vi "Untitled 1.vi"() -> ()   [LabVIEW 2018]
uses:
  <vilib>/imath/engines/lvmath/Plug In/_Char/NIMS_CH_character datatype.ctl
  <vilib>/imath/engines/lvmath2/RunTimeEngine/Managers/WorkSpace/UID Generator.vi
  <vilib>/imath/engines/lvmath2/RunTimeEngine/BuiltInFunctions/zeros/NIMS_V=zeros(I32,I32).vi
  <vilib>/imathl/engines/lvmath/Functions/Error Handling/Create Error.vi
  <vilib>/imath/engines/lvmath2/RunTimeEngine/IndexReplace/NIMS V(S)=S.vi
  <instcachedir>/0/NIMS V(S)=S_420DA4522869420292A92FA3CC108C4E.lvgen/NIMS V(S)=S_420DA4522869420292A92FA3CC108C4E_000.vi
  <vilib>/imath/engines/lvmath2/RunTimeEngine/RangeToken/NIMS_Range_R2 - Float.vi
  <instcachedir>/0/NIMS_Range_R2 - Float_6ECC2DCA6A8F4201A61F790A8BE580A7.lvgen/NIMS_Range_R2 - Float_6ECC2DCA6A8F4201A61F790A8BE580A7_000.vi
  <vilib>/imath/engines/lvmath2/RunTimeEngine/CommandStatement/MC_CommandStatement_break.vi
  <vilib>/imath/engines/lvmath2/RunTimeSupport/NIMS_Error if Not Equal.vi
  <instcachedir>/0/NIMS_Error if Not Equal_C77461FADD9B4AE6B0EA3ED6E3A6D94D.lvgen/NIMS_Error if Not Equal_C77461FADD9B4AE6B0EA3ED6E3A6D94D_000.vi
  <vilib>/imath/engines/lvmath2/RunTimeEngine/IndexRead/NIMS V(S).vi
  <instcachedir>/0/NIMS V(S)_0488751826AF41519A22953C041130DC.lvgen/NIMS V(S)_0488751826AF41519A22953C041130DC_000.vi
  <vilib>/imath/engines/lvmath2/RunTimeEngine/BuiltInFunctions/mod/NIMS_mod_no_size_check.vi
  <instcachedir>/0/NIMS_mod_no_size_check_5393E3382FD241D281EEB71DA286C65B.lvgen/NIMS_mod_no_size_check_5393E3382FD241D281EEB71DA286C65B_001.vi
  <vilib>/imath/engines/lvmath2/RunTimeEngine/ErrorHandling/NIMS_Create Error From Enums.vi
  <vilib>/imath/engines/lvmath2/RunTimeEngine/BuiltInFunctions/histogram/NIMS_[V]=histogram(V).vi
  <vilib>/imath/engines/lvmath2/RunTimeEngine/BuiltInFunctions/max/1 input/NIMS_max(RV).vi
  <instcachedir>/0/NIMS_max(RV)_237633DB1D604D5BA7001287DF3C7957.lvgen/NIMS_max(RV)_237633DB1D604D5BA7001287DF3C7957_002.vi
  <vilib>/imath/engines/lvmath2/RunTimeEngine/RunTimeType/NIMS_RunTimeType_From StrictType (excl LVString).vi
  <instcachedir>/0/NIMS_RunTimeType_From StrictType (excl LVString)_E7E34A65C99947108168652BAD14964D.lvgen/NIMS_RunTimeType_From StrictType (excl LVString)_E7E34A65C99947108168652BAD14964D_001.vi
  <vilib>/imath/engines/lvmath2/RunTimeEngine/LocalVariableDefStatement/MC_LocalVariableDefStatement_Display.vi
  <vilib>/imath/engines/lvmath2/RunTimeEngine/BuiltInFunctions/num_to_str/NIMS_num_to_str(GRowV,I32).vi
  <instcachedir>/0/NIMS_num_to_str(GRowV,I32)_BAB3BCC9D93D469AB30EB0CE4C0C4B02.lvgen/NIMS_num_to_str(GRowV,I32)_BAB3BCC9D93D469AB30EB0CE4C0C4B02_000.vi
  <vilib>/imath/engines/lvmath/Plug In/_Char/NIMS_CH_String to Character Array.vi
  <vilib>/imath/engines/lvmath2/RunTimeEngine/Managers/SymbolTable/Clear UID.vi
  <vilib>/imath/engines/lvmath2/RunTimeEngine/NodeEndStatement/NIMS_NodeEndStatement_Output.vi
  <instcachedir>/0/NIMS_NodeEndStatement_Output_53EC0D466D134D7ABD903AC30B43404B.lvgen/NIMS_NodeEndStatement_Output_53EC0D466D134D7ABD903AC30B43404B_005.vi
  <vilib>/imath/engines/lvmath2/RunTimeEngine/ErrorHandling/NIMS_Finalize Error.vi
  <vilib>/imath/engines/lvmath2/RunTimeEngine/Managers/SymbolTable/NIMS_WorkSpace.lvlib
panel:
  out "m":dbl[](array[numeric])
  out "Histogram of the number":dbl[](graph)
  out "Scatter of uniform random number":dbl[](graph)
  out "Waveform of uniform random number":dbl[](graph)
  in  "first":dbl
  in  "r":dbl
  in  "b":dbl
  in  "M":dbl
  in  "num":dbl
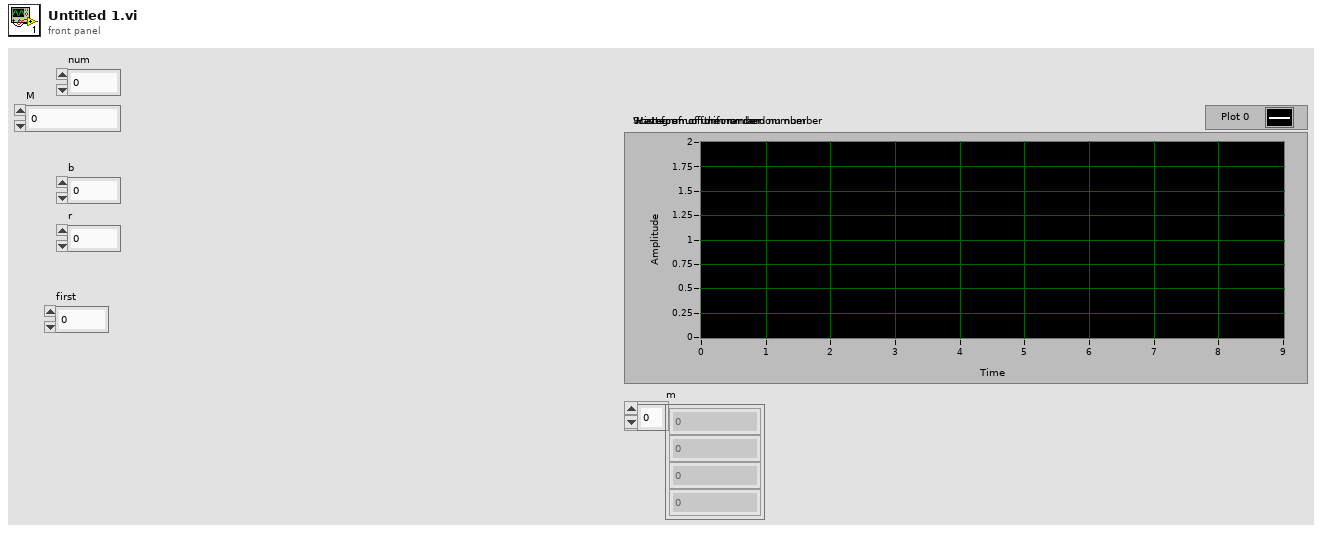
[diagram p1: front panel]
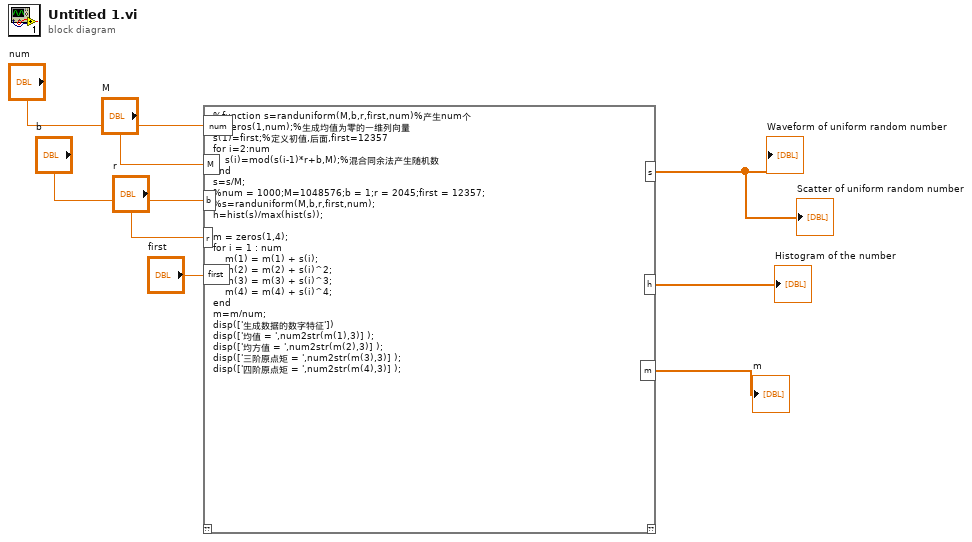
[diagram p0: block diagram]
diagram:
  n1 = mathscript code="%function s=randuniform(M,b,r,first,num)%产生num个\ns=zeros(1,num);%生成均值为零的一维列向量\ns(1)=first;%定义初值,后面,first=12357\nfor i=2:num\n    s(i)=mod(s(i-1)*r+b,M);%混合同余法产生随机数\nend\ns=s/M;\n%num = 1000;M=1048576;b = 1;r = 2045;first = 12357;\n%s=randuniform(M,b,r,first,num);\nh=hist(s)/max(hist(s));\n\nm = zeros(1,4);        \nfor i = 1 : num\n    m(1) = m(1) + s(i);   \n    m(2) = m(2) + s(i)^2; \n    m(3) = m(3) + s(i)^3;  \n    m(4) = m(4) + s(i)^4;  \nend\nm=m/num;\ndisp(['生成数据的数字特征'])\ndisp(['均值 = ',num2str(m(1),3)] );\ndisp(['均方值 = ',num2str(m(2),3)] );\ndisp(['三阶原点矩 = ',num2str(m(3),3)] );\ndisp(['四阶原点矩 = ',num2str(m(4),3)] );"("M"="M", "num"="num", "b"="b", "r"="r", "first"="first") -> ("s"=→"Waveform of uniform random number" →"Scatter of uniform random number":dbl[], "h"=→"Histogram of the number":dbl[], "m"=→"m":dbl[])  [unwired: 1 in, 1 out]
